vi "poly_data_queue_U8.vi"(5 "skip? (F)":bool, 6 "initial queue element (0)":u8, 7 "initialize":bool, 8 "error in":errorcluster caption="Error in (no error)", 9 "queue length (100)":i32=100, 10 "input data point":u8) -> (0 "error out":errorcluster, 1 "eliminated element":u8, 2 "queue":u8[](array[numeric]), 4 "current length":i32)   [LabVIEW 2015]
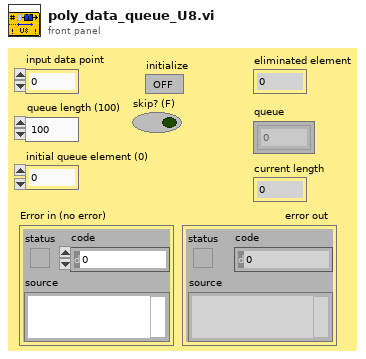
[diagram p1: front panel]
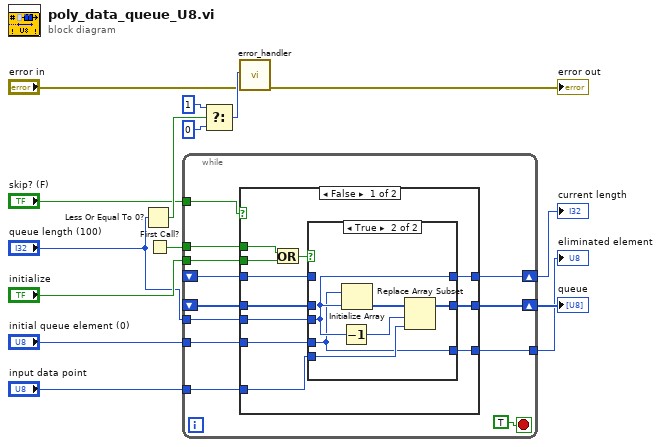
[diagram p0: block diagram]
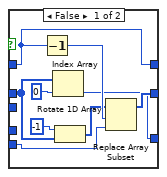
[diagram p2: hidden frame]
diagram:
  n1 = Less Or Equal To 0?(x="queue length (100)") -> (x <= 0?=w7:bool)
  n2 = First Call?() -> (First Call?: T/F=w8:bool)
  n3 = while {
    tunnel: w8 -> [w22]
    shift-left: _ -> [w25]
    shift-right: [w26] -> w14
    shift-left: _ -> [w24]
    shift-right: [w27] -> w15
    tunnel: "initialize" -> [w21]
    tunnel: "input data point" -> [w20]
    tunnel: "initial queue element (0)" -> [w19]
    tunnel: "queue length (100)" -> [w18]
    tunnel: [w17] -> w10
    tunnel: "skip? (F)" -> [w16]
    stop <- TRUE stop-if-true
    n4 = case shown="False" w16 {
      tunnel: [w38 w56] -> w27
      tunnel: [w37 w55] -> w26
      tunnel: w25 -> [w36 w55]
      tunnel: w24 -> [w35 w56]
      tunnel: w22 -> [w34 _]
      tunnel: w21 -> [w32 _]
      tunnel: w20 -> [w31 w54]
      tunnel: w19 -> [w30 _]
      tunnel: w18 -> [w29 _]
      tunnel: [w28 w54] -> w17
      frame False {
        n5 = Or(x=w34, y=w32) -> (x .or. y?=w33:bool)
        n6 = case shown="True" w33 {
          tunnel: [w44 w49] -> w38
          tunnel: [w45 w52] -> w37
          tunnel: w36 -> [w45 _]
          tunnel: w35 -> [w41 _]
          tunnel: w31 -> [w46 w50]
          tunnel: w30 -> [_ w48]
          tunnel: w29 -> [_ w52]
          tunnel: [w39 w48] -> w28
          frame False {
            n7 = Decrement(x=w45) -> (x-1=w43:i32)
            n8 = Index Array(array=w41, index=0 ("Index")) -> (element=w39:u8)
            n9 = Rotate 1D Array(1:w41, 2:i16 -1 ("n")) -> (0:w42:u8[])
            n10 = Replace Array Subset(array=w42, new element=w46, index=w43) -> (w44:u8[])
          }
          frame True {
            n11 = Decrement(x=w52) -> (x-1=w53:i32)
            n12 = Initialize Array(w48, w52) -> (w51:u8[])
            n13 = Replace Array Subset(array=w51, new element=w50, index=w53) -> (w49:u8[])
          }
        }
      }
      frame True {
      }
    }
  }
  "queue" <- w15
  "current length" <- w14
  "eliminated element" <- w10
  n14 = Select(t=1, s=w7, f=0) -> (s? t:f=w4:i32)
  n15 = call "error_handler.vi"("error in (no error)"="error in", "code (0 = no error)"=w4) -> ("error out"=→"error out":errorcluster)  [unwired: 8 in, 1 out]
